vi "Stop_Trigger.vi"(8 "error in (no error)":errorcluster, 9 "Command_Message_in":T1, 11 "DAQ_VI":refnum<vi>) -> (0 "error out":errorcluster, 1 "Command_Message_out":T1)   [LabVIEW 2020]
uses:
  Command_Message.ctl
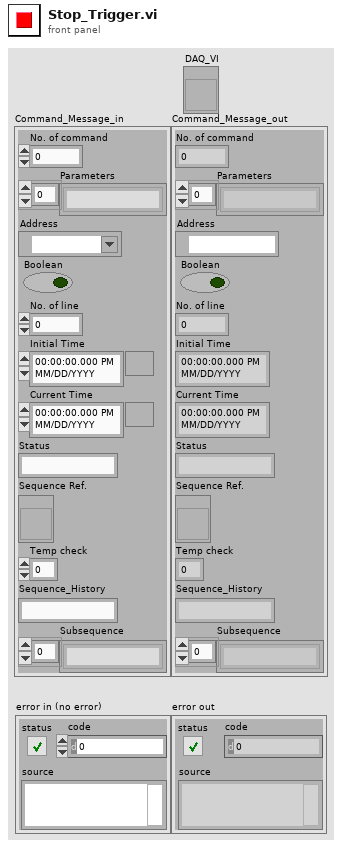
[diagram p1: front panel]
types:
  T1 = typedef "Command_Message.ctl" = cluster{"No. of command":i32, "Parameters":string[], "Address":refnum<visa-resource-name>, "Boolean":bool, "No. of line":i32, "Initial Time":timestamp, "Current Time":timestamp, "Status":string, "Sequence Ref.":refnum<vi>, "Temp check":i32, "Sequence_History":string, "Subsequence":string[]}
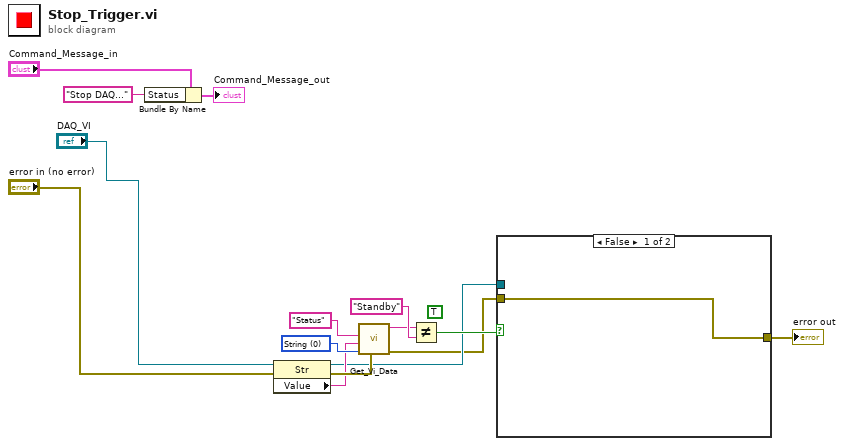
[diagram p0: block diagram]
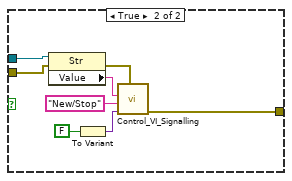
[diagram p2: hidden frame]
diagram:
  (unwired) TRUE
  w12 = u16 0 items=["String", "Double", "Boolean", "Variant"] ("Data Type")
  n1 = Bundle By Name(cluster="Command_Message_in", "Status"="Stop DAQ...") -> (→"Command_Message_out":T1)
  n2 = property on="Property Node" class="Str"(reference="DAQ_VI", error in="error in (no error)") -> (reference out=w3:refnum<vi>, error out=w10:errorcluster, "Value"=w9:string)
  n3 = call "Get_Vi_Data.vi"("error in (no error) 2"=w10, "Data Type"=w12, "VI name"=w9, "Control Name"="Status") -> ("error out"=w2:errorcluster, "Data (String)"=w7:string)  [unwired: 3 in, 3 out]
  n4 = Not Equal?(x=w7, y="Standby") -> (x != y?=w4:bool)
  n5 = case shown="False" w4 {
    tunnel: w3 -> [_ w19]
    tunnel: w2 -> [w16 w18]
    tunnel: [w16 w17] -> w1
    frame False {
    }
    frame True {
      n6 = property on="Property Node" class="Str"(reference=w19, error in=w18) -> (error out=w20:errorcluster, "Value"=w23:string)  [unwired: 1 out]
      n7 = To Variant(anything=FALSE) -> (Variant=w22:variant)
      n8 = call "Control_VI_Signalling.vi"("error in (no error)"=w20, "Input Value"=w22, "Control Name"="New/Stop", "Target VI name"=w23) -> ("error out"=w17:errorcluster)  [unwired: 7 in]
    }
  }
  "error out" <- w1
